vi "GeoData.vi"() -> ()   [LabVIEW 2017] (continued)
County\tH1\n43768\t39059\tOld washington\tOH\tGuernsey County\tH1\n43732\t39059\tCumberland\tOH\tGuernsey County\tH1\n43778\t39059\tSalesville\tOH\tGuernsey County\tH1\n43713\t39059\tBarnesville\tOH\tGuernsey County\tH1\n43722\t39059\tBuffalo\tOH\tGuernsey County\tH1\n43736\t39059\tFairview\tOH\tGuernsey County\tH1\n45013\t39061\tHamilton\tOH\tHamilton County\tH1\n45014\t39061\tFairfield\tOH\tHamilton County\tH1\n45002\t39061\tCleves\tOH\tHamilton County\tH1\n45236\t39061\tCincinnati\tOH\tHamilton County\tH1\n45248\t39061\tCincinnati\tOH\tHamilton County\tH1\n45255\t39061\tCincinnati\tOH\tHamilton County\tH1\n45249\t39061\tCincinnati\tOH\tHamilton County\tH1\n45253\t39061\tCincinnati\tOH\tHamilton County\tH1\n45262\t39061\tCincinnati\tOH\tHamilton County\tH1\n45258\t39061\tCincinnati\tOH\tHamilton County\tH1\n45041\t39061\tMiamitown\tOH\tHamilton County\tH1\n45150\t39061\tMilford\tOH\tHamilton County\tH1\n45069\t39061\tWest chester\tOH\tHamilton County\tH1\n45201\t39061\tCincinnati\tOH\tHamilton County\tH1\n45233\t39061\tCincinnati\tOH\tHamilton County\tH1\n45219\t39061\tCincinnati\tOH\tHamilton County\tH1\n45254\t39061\tCincinnati\tOH\tHamilton County\tH1\n45111\t39061\tCamp dennison\tOH\tHamilton County\tH1\n45263\t39061\tCincinnati\tOH\tHamilton County\tH1\n45208\t39061\tCincinnati\tOH\tHamilton County\tH1\n45211\t39061\tCincinnati\tOH\tHamilton County\tH1\n45204\t39061\tCincinnati\tOH\tHamilton County\tH1\n45226\t39061\tCincinnati\tOH\tHamilton County\tH1\n45227\t39061\tCincinnati\tOH\tHamilton County\tH1\n45229\t39061\tCincinnati\tOH\tHamilton County\tH1\n45220\t39061\tCincinnati\tOH\tHamilton County\tH1\n45235\t39061\tCincinnati\tOH\tHamilton County\tH1\n45030\t39061\tHarrison\tOH\tHamilton County\tH1\n45033\t39061\tHooven\tOH\tHamilton County\tH1\n45206\t39061\tCincinnati\tOH\tHamilton County\tH1\n45212\t39061\tCincinnati\tOH\tHamilton County\tH1\n45213\t39061\tCincinnati\tOH\tHamilton County\tH1\n45247\t39061\tCincinnati\tOH\tHamilton County\tH1\n45224\t39061\tCincinnati\tOH\tHamilton County\tH1\n45238\t39061\tCincinnati\tOH\tHamilton County\tH1\n45230\t39061\tCincinnati\tOH\tHamilton County\tH1\n45052\t39061\tNorth bend\tOH\tHamilton County\tH1\n45202\t39061\tCincinnati\tOH\tHamilton County\tH1\n45215\t39061\tCincinnati\tOH\tHamilton County\tH1\n45242\t39061\tCincinnati\tOH\tHamilton County\tH1\n45251\t39061\tCincinnati\tOH\tHamilton County\tH1\n45217\t39061\tCincinnati\tOH\tHamilton County\tH1\n45232\t39061\tCincinnati\tOH\tHamilton County\tH1\n45001\t39061\tAddyston\tOH\tHamilton County\tH1\n45222\t39061\tCincinnati\tOH\tHamilton County\tH1\n45209\t39061\tCincinnati\tOH\tHamilton County\tH1\n45216\t39061\tCincinnati\tOH\tHamilton County\tH1\n45239\t39061\tCincinnati\tOH\tHamilton County\tH1\n45244\t39061\tCincinnati\tOH\tHamilton County\tH1\n45231\t39061\tCincinnati\tOH\tHamilton County\tH1\n45252\t39061\tCincinnati\tOH\tHamilton County\tH1\n45223\t39061\tCincinnati\tOH\tHamilton County\tH1\n45225\t39061\tCincinnati\tOH\tHamilton County\tH1\n45250\t39061\tCincinnati\tOH\tHamilton County\tH1\n45218\t39061\tCincinnati\tOH\tHamilton County\tH1\n45234\t39061\tCincinnati\tOH\tHamilton County\tH1\n45203\t39061\tCincinnati\tOH\tHamilton County\tH1\n45246\t39061\tCincinnati\tOH\tHamilton County\tH1\n45237\t39061\tCincinnati\tOH\tHamilton County\tH1\n45243\t39061\tCincinnati\tOH\tHamilton County\tH1\n45267\t39061\tCincinnati\tOH\tHamilton County\tH1\n45140\t39061\tLoveland\tOH\tHamilton County\tH1\n45214\t39061\tCincinnati\tOH\tHamilton County\tH1\n45207\t39061\tCincinnati\tOH\tHamilton County\tH1\n45205\t39061\tCincinnati\tOH\tHamilton County\tH1\n45240\t39061\tCincinnati\tOH\tHamilton County\tH1\n45241\t39061\tCincinnati\tOH\tHamilton County\tH1\n45174\t39061\tTerrace park\tOH\tHamilton County\tH1\n45051\t39061\tMount saint joseph\tOH\tHamilton County\tH1\n45810\t39063\tAda\tOH\tHancock County\tH1\n45843\t39063\tForest\tOH\tHancock County\tH1\n45858\t39063\tMc comb\tOH\tHancock County\tH1\n45840\t39063\tFindlay\tOH\tHancock County\tH1\n45867\t39063\tMount blanchard\tOH\tHancock County\tH1\n45877\t39063\tPandora\tOH\tHancock County\tH1\n44802\t39063\tAlvada\tOH\tHancock County\tH1\n43516\t39063\tDeshler\tOH\tHancock County\tH1\n45814\t39063\tArlington\tOH\tHancock County\tH1\n45856\t39063\tLeipsic\tOH\tHancock County\tH1\n45881\t39063\tRawson\tOH\tHancock County\tH1\n44830\t39063\tFostoria\tOH\tHancock County\tH1\n45890\t39063\tVanlue\tOH\tHancock County\tH1\n45817\t39063\tBluffton\tOH\tHancock County\tH1\n45872\t39063\tNorth baltimore\tOH\tHancock County\tH1\n45836\t39063\tDunkirk\tOH\tHancock County\tH1\n45889\t39063\tVan buren\tOH\tHancock County\tH1\n45868\t39063\tMount cory\tOH\tHancock County\tH1\n44817\t39063\tBloomdale\tOH\tHancock County\tH1\n45841\t39063\tJenera\tOH\tHancock County\tH1\n43316\t39063\tCarey\tOH\tHancock County\tH1\n44804\t39063\tArcadia\tOH\tHancock County\tH1\n45839\t39063\tFindlay\tOH\tHancock County\tH1\n45897\t39063\tWilliamstown\tOH\tHancock County\tH1\n45816\t39063\tBenton ridge\tOH\tHancock County\tH1\n45810\t39065\tAda\tOH\tHardin County\tH1\n45843\t39065\tForest\tOH\tHardin County\tH1\n43331\t39065\tLakeview\tOH\tHardin County\tH1\n45850\t39065\tHarrod\tOH\tHardin County\tH1\n43345\t39065\tRidgeway\tOH\tHardin County\tH1\n43310\t39065\tBelle center\tOH\tHardin County\tH1\n43326\t39065\tKenton\tOH\tHardin County\tH1\n43332\t39065\tLa rue\tOH\tHardin County\tH1\n45896\t39065\tWaynesfield\tOH\tHardin County\tH1\n43340\t39065\tMount victory\tOH\tHardin County\tH1\n43347\t39065\tRushsylvania\tOH\tHardin County\tH1\n45859\t39065\tMc guffey\tOH\tHardin County\tH1\n45836\t39065\tDunkirk\tOH\tHardin County\tH1\n45835\t39065\tDola\tOH\tHardin County\tH1\n45841\t39065\tJenera\tOH\tHardin County\tH1\n43346\t39065\tRoundhead\tOH\tHardin County\tH1\n45812\t39065\tAlger\tOH\tHardin County\tH1\n44695\t39067\tBowerston\tOH\tHarrison County\tH1\n43977\t39067\tFlushing\tOH\tHarrison County\tH1\n44699\t39067\tTippecanoe\tOH\tHarrison County\tH1\n43976\t39067\tHopedale\tOH\tHarrison County\tH1\n43988\t39067\tScio\tOH\tHarrison County\tH1\n43907\t39067\tCadiz\tOH\tHarrison County\tH1\n44621\t39067\tDennison\tOH\tHarrison County\tH1\n43983\t39067\tPiedmont\tOH\tHarrison County\tH1\n43974\t39067\tHarrisville\tOH\tHarrison County\tH1\n43981\t39067\tNew athens\tOH\tHarrison County\tH1\n43984\t39067\tNew rumley\tOH\tHarrison County\tH1\n43901\t39067\tAdena\tOH\tHarrison County\tH1\n43973\t39067\tFreeport\tOH\tHarrison County\tH1\n44683\t39067\tUhrichsville\tOH\tHarrison County\tH1\n43986\t39067\tJewett\tOH\tHarrison County\tH1\n44693\t39067\tDeersville\tOH\tHarrison County\tH1\n43950\t39067\tSaint clairsville\tOH\tHarrison County\tH1\n43910\t39067\tBloomingdale\tOH\tHarrison County\tH1\n43527\t39069\tHolgate\tOH\tHenry County\tH1\n43532\t39069\tLiberty center\tOH\tHenry County\tH1\n43548\t39069\tNew bavaria\tOH\tHenry County\tH1\n43510\t39069\tColton\tOH\tHenry County\tH1\n43529\t39069\tHoytville\tOH\tHenry County\tH1\n43515\t39069\tDelta\tOH\tHenry County\tH1\n43516\t39069\tDeshler\tOH\tHenry County\tH1\n43524\t39069\tHamler\tOH\tHenry County\tH1\n45856\t39069\tLeipsic\tOH\tHenry County\tH1\n43535\t39069\tMalinta\tOH\tHenry County\tH1\n43523\t39069\tGrelton\tOH\tHenry County\tH1\n43567\t39069\tWauseon\tOH\tHenry County\tH1\n43512\t39069\tDefiance\tOH\tHenry County\tH1\n43522\t39069\tGrand rapids\tOH\tHenry County\tH1\n43534\t39069\tMc clure\tOH\tHenry County\tH1\n43555\t39069\tRidgeville corners\tOH\tHenry County\tH1\n43502\t39069\tArchbold\tOH\tHenry County\tH1\n43557\t39069\tStryker\tOH\tHenry County\tH1\n43545\t39069\tNapoleon\tOH\tHenry County\tH1\n43511\t39069\tCustar\tOH\tHenry County\tH1\n45660\t39071\tPeebles\tOH\tHighland County\tH1\n45118\t39071\tFayetteville\tOH\tHighland County\tH1\n45172\t39071\tSinking spring\tOH\tHighland County\tH1\n45142\t39071\tLynchburg\tOH\tHighland County\tH1\n45159\t39071\tNew vienna\tOH\tHighland County\tH1\n45697\t39071\tWinchester\tOH\tHighland County\tH1\n45154\t39071\tMount orab\tOH\tHighland County\tH1\n45132\t39071\tHighland\tOH\tHighland County\tH1\n45155\t39071\tMowrystown\tOH\tHighland County\tH1\n45171\t39071\tSardinia\tOH\tHighland County\tH1\n45123\t39071\tGreenfield\tOH\tHighland County\tH1\n45135\t39071\tLeesburg\tOH\tHighland County\tH1\n45679\t39071\tSeaman\tOH\tHighland County\tH1\n45133\t39071\tHillsboro\tOH\tHighland County\tH1\n45612\t39071\tBainbridge\tOH\tHighland County\tH1\n45654\t39073\tNew plymouth\tOH\tHocking County\tH1\n43158\t39073\tUnion furnace\tOH\tHocking County\tH1\n43155\t39073\tSugar grove\tOH\tHocking County\tH1\n43766\t39073\tNew straitsville\tOH\tHocking County\tH1\n43107\t39073\tBremen\tOH\tHocking County\tH1\n45622\t39073\tCreola\tOH\tHocking County\tH1\n43149\t39073\tRockbridge\tOH\tHocking County\tH1\n43102\t39073\tAmanda\tOH\tHocking County\tH1\n45732\t39073\tGlouster\tOH\tHocking County\tH1\n43127\t39073\tHaydenville\tOH\tHocking County\tH1\n43144\t39073\tMurray city\tOH\tHocking County\tH1\n43130\t39073\tLancaster\tOH\tHocking County\tH1\n43138\t39073\tLogan\tOH\tHocking County\tH1\n45764\t39073\tNelsonville\tOH\tHocking County\tH1\n43111\t39073\tCarbon hill\tOH\tHocking County\tH1\n43152\t39073\tSouth bloomingville\tOH\tHocking County\tH1\n43135\t39073\tLaurelville\tOH\tHocking County\tH1\n44660\t39075\tMount hope\tOH\tHolmes County\tH1\n44661\t39075\tNashville\tOH\tHolmes County\tH1\n44617\t39075\tCharm\tOH\tHolmes County\tH1\n44627\t39075\tFredericksburg\tOH\tHolmes County\tH1\n44690\t39075\tWinesburg\tOH\tHolmes County\tH1\n44637\t39075\tKillbuck\tOH\tHolmes County\tH1\n44610\t39075\tBerlin\tOH\tHolmes County\tH1\n44681\t39075\tSugarcreek\tOH\tHolmes County\tH1\n44676\t39075\tShreve\tOH\tHolmes County\tH1\n44689\t39075\tWilmot\tOH\tHolmes County\tH1\n44654\t39075\tMillersburg\tOH\tHolmes County\tH1\n44624\t39075\tDundee\tOH\tHolmes County\tH1\n43804\t39075\tBaltic\tOH\tHolmes County\tH1\n44628\t39075\tGlenmont\tOH\tHolmes County\tH1\n44687\t39075\tWalnut creek\tOH\tHolmes County\tH1\n44611\t39075\tBig prairie\tOH\tHolmes County\tH1\n44842\t39075\tLoudonville\tOH\tHolmes County\tH1\n43006\t39075\tBrinkhaven\tOH\tHolmes County\tH1\n44633\t39075\tHolmesville\tOH\tHolmes County\tH1\n44638\t39075\tLakeville\tOH\tHolmes County\tH1\n44847\t39077\tMonroeville\tOH\tHuron County\tH1\n44889\t39077\tWakeman\tOH\tHuron County\tH1\n44837\t39077\tGreenwich\tOH\tHuron County\tH1\n44878\t39077\tShiloh\tOH\tHuron County\tH1\n44826\t39077\tCollins\tOH\tHuron County\tH1\n44890\t39077\tWillard\tOH\tHuron County\tH1\n44851\t39077\tNew london\tOH\tHuron County\tH1\n44807\t39077\tAttica\tOH\tHuron County\tH1\n44811\t39077\tBellevue\tOH\tHuron County\tH1\n44865\t39077\tPlymouth\tOH\tHuron County\tH1\n44850\t39077\tNew haven\tOH\tHuron County\tH1\n44888\t39077\tWillard\tOH\tHuron County\tH1\n44855\t39077\tNorth fairfield\tOH\tHuron County\tH1\n44854\t39077\tNew washington\tOH\tHuron County\tH1\n44846\t39077\tMilan\tOH\tHuron County\tH1\n44857\t39077\tNorwalk\tOH\tHuron County\tH1\n45601\t39079\tChillicothe\tOH\tJackson County\tH1\n45621\t39079\tCoalton\tOH\tJackson County\tH1\n45653\t39079\tMinford\tOH\tJackson County\tH1\n45686\t39079\tVinton\tOH\tJackson County\tH1\n45656\t39079\tOak hill\tOH\tJackson County\tH1\n45634\t39079\tHamden\tOH\tJackson County\tH1\n45640\t39079\tJackson\tOH\tJackson County\tH1\n45672\t39079\tRay\tOH\tJackson County\tH1\n45682\t39079\tSouth webster\tOH\tJackson County\tH1\n45692\t39079\tWellston\tOH\tJackson County\tH1\n45685\t39079\tThurman\tOH\tJackson County\tH1\n45613\t39079\tBeaver\tOH\tJackson County\tH1\n43917\t39081\tDillonvale\tOH\tJefferson County\tH1\n43964\t39081\tToronto\tOH\tJefferson County\tH1\n43939\t39081\tMount pleasant\tOH\tJefferson County\tH1\n43943\t39081\tRayland\tOH\tJefferson County\tH1\n43907\t39081\tCadiz\tOH\tJefferson County\tH1\n43908\t39081\tBergholz\tOH\tJefferson County\tH1\n43944\t39081\tRichmond\tOH\tJefferson County\tH1\n43930\t39081\tHammondsville\tOH\tJefferson County\tH1\n43926\t39081\tEmpire\tOH\tJefferson County\tH1\n43945\t39081\tSalineville\tOH\tJefferson County\tH1\n43952\t39081\tSteubenville\tOH\tJefferson County\tH1\n43932\t39081\tIrondale\tOH\tJefferson County\tH1\n43963\t39081\tTiltonsville\tOH\tJefferson County\tH1\n43948\t39081\tSmithfield\tOH\tJefferson County\tH1\n43901\t39081\tAdena\tOH\tJefferson County\tH1\n43953\t39081\tSteubenville\tOH\tJefferson County\tH1\n43903\t39081\tAmsterdam\tOH\tJefferson County\tH1\n43941\t39081\tPiney fork\tOH\tJefferson County\tH1\n43925\t39081\tEast springfield\tOH\tJefferson County\tH1\n43938\t39081\tMingo junction\tOH\tJefferson County\tH1\n43971\t39081\tYorkville\tOH\tJefferson County\tH1\n43913\t39081\tBrilliant\tOH\tJefferson County\tH1\n43961\t39081\tStratton\tOH\tJefferson County\tH1\n43970\t39081\tWolf run\tOH\tJefferson County\tH1\n43910\t39081\tBloomingdale\tOH\tJefferson County\tH1\n43080\t39083\tUtica\tOH\tKnox County\tH1\n43050\t39083\tMount vernon\tOH\tKnox County\tH1\n44822\t39083\tButler\tOH\tKnox County\tH1\n43028\t39083\tHoward\tOH\tKnox County\tH1\n43022\t39083\tGambier\tOH\tKnox County\tH1\n44628\t39083\tGlenmont\tOH\tKnox County\tH1\n43005\t39083\tBladensburg\tOH\tKnox County\tH1\n44842\t39083\tLoudonville\tOH\tKnox County\tH1\n43844\t39083\tWarsaw\tOH\tKnox County\tH1\n43822\t39083\tFrazeysburg\tOH\tKnox County\tH1\n43006\t39083\tBrinkhaven\tOH\tKnox County\tH1\n43048\t39083\tMount liberty\tOH\tKnox County\tH1\n43014\t39083\tDanville\tOH\tKnox County\tH1\n43037\t39083\tMartinsburg\tOH\tKnox County\tH1\n44813\t39083\tBellville\tOH\tKnox County\tH1\n43019\t39083\tFredericktown\tOH\tKnox County\tH1\n43011\t39083\tCenterburg\tOH\tKnox County\tH1\n43843\t39083\tWalhonding\tOH\tKnox County\tH1\n44041\t39085\tGeneva\tOH\tLake County\tH1\n44086\t39085\tThompson\tOH\tLake County\tH1\n44024\t39085\tChardon\tOH\tLake County\tH1\n44060\t39085\tMentor\tOH\tLake County\tH1\n44094\t39085\tWilloughby\tOH\tLake County\tH1\n44092\t39085\tWickliffe\tOH\tLake County\tH1\n44095\t39085\tEastlake\tOH\tLake County\tH1\n44061\t39085\tMentor\tOH\tLake County\tH1\n44096\t39085\tWilloughby\tOH\tLake County\tH1\n44132\t39085\tEuclid\tOH\tLake County\tH1\n44057\t39085\tMadison\tOH\tLake County\tH1\n44081\t39085\tPerry\tOH\tLake County\tH1\n44077\t39085\tPainesville\tOH\tLake County\tH1\n44045\t39085\tGrand river\tOH\tLake County\tH1\n45623\t39087\tCrown city\tOH\tLawrence County\tH1\n45658\t39087\tPatriot\tOH\tLawrence County\tH1\n45638\t39087\tIronton\tOH\tLawrence County\tH1\n45669\t39087\tProctorville\tOH\tLawrence County\tH1\n45688\t39087\tWaterloo\tOH\tLawrence County\tH1\n45629\t39087\tFranklin furnace\tOH\tLawrence County\tH1\n45696\t39087\tWillow wood\tOH\tLawrence County\tH1\n45659\t39087\tPedro\tOH\tLawrence County\tH1\n45656\t39087\tOak hill\tOH\tLawrence County\tH1\n45645\t39087\tKitts hill\tOH\tLawrence County\tH1\n45619\t39087\tChesapeake\tOH\tLawrence County\tH1\n45682\t39087\tSouth webster\tOH\tLawrence County\tH1\n45675\t39087\tRock camp\tOH\tLawrence County\tH1\n45680\t39087\tSouth point\tOH\tLawrence County\tH1\n45678\t39087\tScottown\tOH\tLawrence County\tH1\n43076\t39089\tThornville\tOH\tLicking County\tH1\n43080\t39089\tUtica\tOH\tLicking County\tH1\n43050\t39089\tMount vernon\tOH\tLicking County\tH1\n43023\t39089\tGranville\tOH\tLicking County\tH1\n43746\t39089\tHopewell\tOH\tLicking County\tH1\n43031\t39089\tJohnstown\tOH\tLicking County\tH1\n43739\t39089\tGlenford\tOH\tLicking County\tH1\n43004\t39089\tBlacklick\tOH\tLicking County\tH1\n43018\t39089\tEtna\tOH\tLicking County\tH1\n43760\t39089\tMount perry\tOH\tLicking County\tH1\n43030\t39089\tJacksontown\tOH\tLicking County\tH1\n43105\t39089\tBaltimore\tOH\tLicking County\tH1\n43147\t39089\tPickerington\tOH\tLicking County\tH1\n43740\t39089\tGratiot\tOH\tLicking County\tH1\n43054\t39089\tNew albany\tOH\tLicking County\tH1\n43046\t39089\tMillersport\tOH\tLicking County\tH1\n43830\t39089\tNashport\tOH\tLicking County\tH1\n43025\t39089\tHebron\tOH\tLicking County\tH1\n43033\t39089\tKirkersville\tOH\tLicking County\tH1\n43068\t39089\tReynoldsburg\tOH\tLicking County\tH1\n43055\t39089\tNewark\tOH\tLicking County\tH1\n43056\t39089\tHeath\tOH\tLicking County\tH1\n43013\t39089\tCroton\tOH\tLicking County\tH1\n43822\t39089\tFrazeysburg\tOH\tLicking County\tH1\n43027\t39089\tHomer\tOH\tLicking County\tH1\n43071\t39089\tSaint louisville\tOH\tLicking County\tH1\n43074\t39089\tSunbury\tOH\tLicking County\tH1\n43062\t39089\tPataskala\tOH\tLicking County\tH1\n43008\t39089\tBuckeye lake\tOH\tLicking County\tH1\n43058\t39089\tNewark\tOH\tLicking County\tH1\n43011\t39089\tCenterburg\tOH\tLicking County\tH1\n43001\t39089\tAlexandria\tOH\tLicking County\tH1\n43721\t39089\tBrownsville\tOH\tLicking County\tH1\n43073\t39089\tSummit station\tOH\tLicking County\tH1\n43331\t39091\tLakeview\tOH\tLogan County\tH1\n43311\t39091\tBellefontaine\tOH\tLogan County\tH1\n43319\t39091\tEast liberty\tOH\tLogan County\tH1\n43348\t39091\tRussells point\tOH\tLogan County\tH1\n43345\t39091\tRidgeway\tOH\tLogan County\tH1\n43310\t39091\tBelle center\tOH\tLogan County\tH1\n43357\t39091\tWest liberty\tOH\tLogan County\tH1\n43067\t39091\tRaymond\tOH\tLogan County\tH1\n45895\t39091\tWapakoneta\tOH\tLogan County\tH1\n43060\t39091\tNorth lewisburg\tOH\tLogan County\tH1\n43347\t39091\tRushsylvania\tOH\tLogan County\tH1\n43336\t39091\tMiddleburg\tOH\tLogan County\tH1\n43358\t39091\tWest mansfield\tOH\tLogan County\tH1\n43333\t39091\tLewistown\tOH\tLogan County\tH1\n43343\t39091\tQuincy\tOH\tLogan County\tH1\n43318\t39091\tDe graff\tOH\tLogan County\tH1\n43360\t39091\tZanesfield\tOH\tLogan County\tH1\n45334\t39091\tJackson center\tOH\tLogan County\tH1\n43324\t39091\tHuntsville\tOH\tLogan County\tH1\n44275\t39093\tSpencer\tOH\tLorain County\tH1\n44074\t39093\tOberlin\tOH\tLorain County\tH1\n44859\t39093\tNova\tOH\tLorain County\tH1\n44012\t39093\tAvon lake\tOH\tLorain County\tH1\n44256\t39093\tMedina\tOH\tLorain County\tH1\n44889\t39093\tWakeman\tOH\tLorain County\tH1\n44044\t39093\tGrafton\tOH\tLorain County\tH1\n44039\t39093\tNorth ridgeville\tOH\tLorain County\tH1\n44001\t39093\tAmherst\tOH\tLorain County\tH1\n44052\t39093\tLorain\tOH\tLorain County\tH1\n44851\t39093\tNew london\tOH\tLorain County\tH1\n44049\t39093\tKipton\tOH\tLorain County\tH1\n44011\t39093\tAvon\tOH\tLorain County\tH1\n44280\t39093\tValley city\tOH\tLorain County\tH1\n44090\t39093\tWellington\tOH\tLorain County\tH1\n44880\t39093\tSullivan\tOH\tLorain County\tH1\n44036\t39093\tElyria\tOH\tLorain County\tH1\n44035\t39093\tElyria\tOH\tLorain County\tH1\n44053\t39093\tLorain\tOH\tLorain County\tH1\n44028\t39093\tColumbia station\tOH\tLorain County\tH1\n44253\t39093\tLitchfield\tOH\tLorain County\tH1\n44089\t39093\tVermilion\tOH\tLorain County\tH1\n44054\t39093\tSheffield lake\tOH\tLorain County\tH1\n44050\t39093\tLagrange\tOH\tLorain County\tH1\n44055\t39093\tLorain\tOH\tLorain County\tH1\n43612\t39095\tToledo\tOH\tLucas County\tH1\n43606\t39095\tToledo\tOH\tLucas County\tH1\n43571\t39095\tWhitehouse\tOH\tLucas County\tH1\n43609\t39095\tToledo\tOH\tLucas County\tH1\n43532\t39095\tLiberty center\tOH\tLucas County\tH1\n43504\t39095\tBerkey\tOH\tLucas County\tH1\n43547\t39095\tNeapolis\tOH\tLucas County\tH1\n43434\t39095\tHarbor view\tOH\tLucas County\tH1\n43615\t39095\tToledo\tOH\tLucas County\tH1\n43623\t39095\tToledo\tOH\tLucas County\tH1\n43560\t39095\tSylvania\tOH\tLucas County\tH1\n43619\t39095\tNorthwood\tOH\tLucas County\tH1\n43537\t39095\tMaumee\tOH\tLucas County\tH1\n43445\t39095\tMartin\tOH\tLucas County\tH1\n43601\t39095\tToledo\tOH\tLucas County\tH1\n43656\t39095\tToledo\tOH\tLucas County\tH1\n43558\t39095\tSwanton\tOH\tLucas County\tH1\n43528\t39095\tHolland\tOH\tLucas County\tH1\n43635\t39095\tToledo\tOH\tLucas County\tH1\n43659\t39095\tToledo\tOH\tLucas County\tH1\n43657\t39095\tToledo\tOH\tLucas County\tH1\n43611\t39095\tToledo\tOH\tLucas County\tH1\n43614\t39095\tToledo\tOH\tLucas County\tH1\n43604\t39095\tToledo\tOH\tLucas County\tH1\n43666\t39095\tToledo\tOH\tLucas County\tH1\n43667\t39095\tToledo\tOH\tLucas County\tH1\n43613\t39095\tToledo\tOH\tLucas County\tH1\n43620\t39095\tToledo\tOH\tLucas County\tH1\n43617\t39095\tToledo\tOH\tLucas County\tH1\n43412\t39095\tCurtice\tOH\tLucas County\tH1\n43522\t39095\tGrand rapids\tOH\tLucas County\tH1\n43661\t39095\tToledo\tOH\tLucas County\tH1\n43605\t39095\tToledo\tOH\tLucas County\tH1\n43607\t39095\tToledo\tOH\tLucas County\tH1\n43616\t39095\tOregon\tOH\tLucas County\tH1\n43566\t39095\tWaterville\tOH\tLucas County\tH1\n43608\t39095\tToledo\tOH\tLucas County\tH1\n45348\t39095\tNew weston\tOH\tLucas County\tH1\n43660\t39095\tToledo\tOH\tLucas County\tH1\n43652\t39095\tToledo\tOH\tLucas County\tH1\n43542\t39095\tMonclova\tOH\tLucas County\tH1\n43610\t39095\tToledo\tOH\tLucas County\tH1\n43064\t39097\tPlain city\tOH\tMadison County\tH1\n43026\t39097\tHilliard\tOH\tMadison County\tH1\n43029\t39097\tIrwin\tOH\tMadison County\tH1\n45369\t39097\tSouth vienna\tOH\tMadison County\tH1\n43151\t39097\tSedalia\tOH\tMadison County\tH1\n43123\t39097\tGrove city\tOH\tMadison County\tH1\n43162\t39097\tWest jefferson\tOH\tMadison County\tH1\n43140\t39097\tLondon\tOH\tMadison County\tH1\n43143\t39097\tMount sterling\tOH\tMadison County\tH1\n43153\t39097\tSouth solon\tOH\tMadison County\tH1\n43119\t39097\tGalloway\tOH\tMadison County\tH1\n43044\t39097\tMechanicsburg\tOH\tMadison County\tH1\n43146\t39097\tOrient\tOH\tMadison County\tH1\n44512\t39099\tYoungstown\tOH\tMahoning County\tH1\n44451\t39099\tNorth jackson\tOH\tMahoning County\tH1\n44501\t39099\tYoungstown\tOH\tMahoning County\tH1\n44449\t39099\tNorth benton\tOH\tMahoning County\tH1\n44454\t39099\tPetersburg\tOH\tMahoning County\tH1\n44416\t39099\tEllsworth\tOH\tMahoning County\tH1\n44437\t39099\tMc donald\tOH\tMahoning County\tH1\n44460\t39099\tSalem\tOH\tMahoning County\tH1\n44408\t39099\tColumbiana\tOH\tMahoning County\tH1\n44511\t39099\tYoungstown\tOH\tMahoning County\tH1\n44514\t39099\tYoungstown\tOH\tMahoning County\tH1\n44452\t39099\tNorth lima\tOH\tMahoning County\tH1\n44405\t39099\tCampbell\tOH\tMahoning County\tH1\n44504\t39099\tYoungstown\tOH\tMahoning County\tH1\n44436\t39099\tLowellville\tOH\tMahoning County\tH1\n44506\t39099\tYoungstown\tOH\tMahoning County\tH1\n44422\t39099\tGreenford\tOH\tMahoning County\tH1\n44471\t39099\tStruthers\tOH\tMahoning County\tH1\n44507\t39099\tYoungstown\tOH\tMahoning County\tH1\n44503\t39099\tYoungstown\tOH\tMahoning County\tH1\n44481\t39099\tWarren\tOH\tMahoning County\tH1\n44406\t39099\tCanfield\tOH\tMahoning County\tH1\n44515\t39099\tYoungstown\tOH\tMahoning County\tH1\n44509\t39099\tYoungstown\tOH\tMahoning County\tH1\n44490\t39099\tWashingtonville\tOH\tMahoning County\tH1\n44443\t39099\tNew springfield\tOH\tMahoning County\tH1\n44442\t39099\tNew middletown\tOH\tMahoning County\tH1\n44601\t39099\tAlliance\tOH\tMahoning County\tH1\n44672\t39099\tSebring\tOH\tMahoning County\tH1\n44510\t39099\tYoungstown\tOH\tMahoning County\tH1\n44513\t39099\tYoungstown\tOH\tMahoning County\tH1\n44412\t39099\tDiamond\tOH\tMahoning County\tH1\n44555\t39099\tYoungstown\tOH\tMahoning County\tH1\n44425\t39099\tHubbard\tOH\tMahoning County\tH1\n44440\t39099\tMineral ridge\tOH\tMahoning County\tH1\n44401\t39099\tBerlin center\tOH\tMahoning County\tH1\n44429\t39099\tLake milton\tOH\tMahoning County\tH1\n44502\t39099\tYoungstown\tOH\tMahoning County\tH1\n44505\t39099\tYoungstown\tOH\tMahoning County\tH1\n44619\t39099\tDamascus\tOH\tMahoning County\tH1\n44444\t39099\tNewton falls\tOH\tMahoning County\tH1\n44609\t39099\tBeloit\tOH\tMahoning County\tH1\n45843\t39101\tForest\tOH\tMarion County\tH1\n44849\t39101\tNevada\tOH\tMarion County\tH1\n43344\t39101\tRichwood\tOH\tMarion County\tH1\n43326\t39101\tKenton\tOH\tMarion County\tH1\n43332\t39101\tLa rue\tOH\tMarion County\tH1\n43314\t39101\tCaledonia\tOH\tMarion County\tH1\n43337\t39101\tMorral\tOH\tMarion County\tH1\n43302\t39101\tMarion\tOH\tMarion County\tH1\n43315\t39101\tCardington\tOH\tMarion County\tH1\n43341\t39101\tNew bloomington\tOH\tMarion County\tH1\n43322\t39101\tGreen camp\tOH\tMarion County\tH1\n43342\t39101\tProspect\tOH\tMarion County\tH1\n44833\t39101\tGalion\tOH\tMarion County\tH1\n43323\t39101\tHarpster\tOH\tMarion County\tH1\n43356\t39101\tWaldo\tOH\tMarion County\tH1\n44275\t39103\tSpencer\tOH\tMedina County\tH1\n44258\t39103\tMedina\tOH\tMedina County\tH1\n44256\t39103\tMedina\tOH\tMedina County\tH1\n44287\t39103\tWest salem\tOH\tMedina County\tH1\n44251\t39103\tWestfield center\tOH\tMedina County\tH1\n44235\t39103\tHomerville\tOH\tMedina County\tH1\n44215\t39103\tChippewa lake\tOH\tMedina County\tH1\n44274\t39103\tSharon center\tOH\tMedina County\tH1\n44233\t39103\tHinckley\tOH\tMedina County\tH1\n44217\t39103\tCreston\tOH\tMedina County\tH1\n44044\t39103\tGrafton\tOH\tMedina County\tH1\n44230\t39103\tDoylestown\tOH\tMedina County\tH1\n44212\t39103\tBrunswick\tOH\tMedina County\tH1\n44254\t39103\tLodi\tOH\tMedina County\tH1\n44273\t39103\tSeville\tOH\tMedina County\tH1\n44280\t39103\tValley city\tOH\tMedina County\tH1\n44090\t39103\tWellington\tOH\tMedina County\tH1\n44880\t39103\tSullivan\tOH\tMedina County\tH1\n44149\t39103\tStrongsville\tOH\tMedina County\tH1\n44214\t39103\tBurbank\tOH\tMedina County\tH1\n44281\t39103\tWadsworth\tOH\tMedina County\tH1\n44333\t39103\tAkron\tOH\tMedina County\tH1\n44321\t39103\tAkron\tOH\tMedina County\tH1\n44028\t39103\tColumbia station\tOH\tMedina County\tH1\n44203\t39103\tBarberton\tOH\tMedina County\tH1\n44270\t39103\tRittman\tOH\tMedina County\tH1\n44253\t39103\tLitchfield\tOH\tMedina County\tH1\n45723\t39105\tCoolville\tOH\tMeigs County\tH1\n45770\t39105\tPortland\tOH\tMeigs County\tH1\n45720\t39105\tChester\tOH\tMeigs County\tH1\n45776\t39105\tShade\tOH\tMeigs County\tH1\n45769\t39105\tPomeroy\tOH\tMeigs County\tH1\n45771\t39105\tRacine\tOH\tMeigs County\tH1\n45741\t39105\tLangsville\tOH\tMeigs County\tH1\n45760\t39105\tMiddleport\tOH\tMeigs County\tH1\n45614\t39105\tBidwell\tOH\tMeigs County\tH1\n45775\t39105\tRutland\tOH\tMeigs County\tH1\n45686\t39105\tVinton\tOH\tMeigs County\tH1\n45735\t39105\tGuysville\tOH\tMeigs County\tH1\n45783\t39105\tTuppers plains\tOH\tMeigs County\tH1\n45710\t39105\tAlbany\tOH\tMeigs County\tH1\n45743\t39105\tLong bottom\tOH\tMeigs County\tH1\n45772\t39105\tReedsville\tOH\tMeigs County\tH1\n45779\t39105\tSyracuse\tOH\tMeigs County\tH1\n45620\t39105\tCheshire\tOH\tMeigs County\tH1\n45865\t39107\tMinster\tOH\tMercer County\tH1\n45862\t39107\tMendon\tOH\tMercer County\tH1\n45860\t39107\tMaria stein\tOH\tMercer County\tH1\n45883\t39107\tSaint henry\tOH\tMercer County\tH1\n45882\t39107\tRockford\tOH\tMercer County\tH1\n45826\t39107\tChickasaw\tOH\tMercer County\tH1\n45822\t39107\tCelina\tOH\tMercer County\tH1\n45898\t39107\tWillshire\tOH\tMercer County\tH1\n45869\t39107\tNew bremen\tOH\tMercer County\tH1\n45388\t39107\tYorkshire\tOH\tMercer County\tH1\n45894\t39107\tVenedocia\tOH\tMercer County\tH1\n45885\t39107\tSaint marys\tOH\tMercer County\tH1\n45887\t39107\tSpencerville\tOH\tMercer County\tH1\n45846\t39107\tFort recovery\tOH\tMercer County\tH1\n45348\t39107\tNew weston\tOH\tMercer County\tH1\n45828\t39107\tColdwater\tOH\tMercer County\tH1\n45845\t39107\tFort loramie\tOH\tMercer County\tH1\n45310\t39107\tBurkettsville\tOH\tMercer County\tH1\n45866\t39107\tMontezuma\tOH\tMercer County\tH1\n45371\t39109\tTipp city\tOH\tMiami County\tH1\n45383\t39109\tWest milton\tOH\tMiami County\tH1\n45361\t39109\tPotsdam\tOH\tMiami County\tH1\n45374\t39109\tTroy\tOH\tMiami County\tH1\n45304\t39109\tArcanum\tOH\tMiami County\tH1\n45337\t39109\tLaura\tOH\tMiami County\tH1\n45326\t39109\tFletcher\tOH\tMiami County\tH1\n45317\t39109\tConover\tOH\tMiami County\tH1\n45318\t39109\tCovington\tOH\tMiami County\tH1\n45424\t39109\tDayton\tOH\tMiami County\tH1\n45308\t39109\tBradford\tOH\tMiami County\tH1\n45322\t39109\tEnglewood\tOH\tMiami County\tH1\n45344\t39109\tNew carlisle\tOH\tMiami County\tH1\n45339\t39109\tLudlow falls\tOH\tMiami County\tH1\n45373\t39109\tTroy\tOH\tMiami County\tH1\n45365\t39109\tSidney\tOH\tMiami County\tH1\n45312\t39109\tCasstown\tOH\tMiami County\tH1\n45356\t39109\tPiqua\tOH\tMiami County\tH1\n45359\t39109\tPleasant hill\tOH\tMiami County\tH1\n43793\t39111\tWoodsfield\tOH\tMonroe County\tH1\n43942\t39111\tPowhatan point\tOH\tMonroe County\tH1\n43946\t39111\tSardis\tOH\tMonroe County\tH1\n43754\t39111\tLewisville\tOH\tMonroe County\tH1\n43915\t39111\tClarington\tOH\tMonroe County\tH1\n43716\t39111\tBeallsville\tOH\tMonroe County\tH1\n45767\t39111\tNew matamoras\tOH\tMonroe County\tH1\n45734\t39111\tGraysville\tOH\tMonroe County\tH1\n43914\t39111\tCameron\tOH\tMonroe County\tH1\n43773\t39111\tQuaker city\tOH\tMonroe County\tH1\n43747\t39111\tJerusalem\tOH\tMonroe County\tH1\n43788\t39111\tSummerfield\tOH\tMonroe County\tH1\n45745\t39111\tLower salem\tOH\tMonroe County\tH1\n43786\t39111\tStafford\tOH\tMonroe County\tH1\n43752\t39111\tLaings\tOH\tMonroe County\tH1\n43931\t39111\tHannibal\tOH\tMonroe County\tH1\n43757\t39111\tMalaga\tOH\tMonroe County\tH1\n45789\t39111\tWingett run\tOH\tMonroe County\tH1\n45005\t39113\tFranklin\tOH\tMontgomery County\tH1\n45342\t39113\tMiamisburg\tOH\tMontgomery County\tH1\n45315\t39113\tClayton\tOH\tMontgomery County\tH1\n45371\t39113\tTipp city\tOH\tMontgomery County\tH1\n45440\t39113\tDayton\tOH\tMontgomery County\tH1\n45430\t39113\tDayton\tOH\tMontgomery County\tH1\n45345\t39113\tNew lebanon\tOH\tMontgomery County\tH1\n45343\t39113\tMiamisburg\tOH\tMontgomery County\tH1\n45490\t39113\tDayton\tOH\tMontgomery County\tH1\n45354\t39113\tPhillipsburg\tOH\tMontgomery County\tH1\n45377\t39113\tVandalia\tOH\tMontgomery County\tH1\n45415\t39113\tDayton\tOH\tMontgomery County\tH1\n45401\t39113\tDayton\tOH\tMontgomery County\tH1\n45439\t39113\tDayton\tOH\tMontgomery County\tH1\n45416\t39113\tDayton\tOH\tMontgomery County\tH1\n45428\t39113\tDayton\tOH\tMontgomery County\tH1\n45066\t39113\tSpringboro\tOH\tMontgomery County\tH1\n45338\t39113\tLewisburg\tOH\tMontgomery County\tH1\n45409\t39113\tDayton\tOH\tMontgomery County\tH1\n45433\t39113\tDayton\tOH\tMontgomery County\tH1\n45309\t39113\tBrookville\tOH\tMontgomery County\tH1\n45327\t39113\tGermantown\tOH\tMontgomery County\tH1\n45403\t39113\tDayton\tOH\tMontgomery County\tH1\n45406\t39113\tDayton\tOH\tMontgomery County\tH1\n45429\t39113\tDayton\tOH\tMontgomery County\tH1\n45381\t39113\tWest alexandria\tOH\tMontgomery County\tH1\n45423\t39113\tDayton\tOH\tMontgomery County\tH1\n45422\t39113\tDayton\tOH\tMontgomery County\tH1\n45417\t39113\tDayton\tOH\tMontgomery County\tH1\n45419\t39113\tDayton\tOH\tMontgomery County\tH1\n45424\t39113\tDayton\tOH\tMontgomery County\tH1\n45431\t39113\tDayton\tOH\tMontgomery County\tH1\n45449\t39113\tDayton\tOH\tMontgomery County\tH1\n45322\t39113\tEnglewood\tOH\tMontgomery County\tH1\n45405\t39113\tDayton\tOH\tMontgomery County\tH1\n45414\t39113\tDayton\tOH\tMontgomery County\tH1\n45344\t39113\tNew carlisle\tOH\tMontgomery County\tH1\n45420\t39113\tDayton\tOH\tMontgomery County\tH1\n45378\t39113\tVerona\tOH\tMontgomery County\tH1\n45042\t39113\tMiddletown\tOH\tMontgomery County\tH1\n45402\t39113\tDayton\tOH\tMontgomery County\tH1\n45404\t39113\tDayton\tOH\tMontgomery County\tH1\n45410\t39113\tDayton\tOH\tMontgomery County\tH1\n45426\t39113\tDayton\tOH\tMontgomery County\tH1\n45413\t39113\tDayton\tOH\tMontgomery County\tH1\n45458\t39113\tDayton\tOH\tMontgomery County\tH1\n45475\t39113\tDayton\tOH\tMontgomery County\tH1\n45437\t39113\tDayton\tOH\tMontgomery County\tH1\n45469\t39113\tDayton\tOH\tMontgomery County\tH1\n45470\t39113\tDayton\tOH\tMontgomery County\tH1\n45448\t39113\tDayton\tOH\tMontgomery County\tH1\n45325\t39113\tFarmersville\tOH\tMontgomery County\tH1\n45432\t39113\tDayton\tOH\tMontgomery County\tH1\n45441\t39113\tDayton\tOH\tMontgomery County\tH1\n45459\t39113\tDayton\tOH\tMontgomery County\tH1\n43787\t39115\tStockport\tOH\tMorgan County\tH1\n45715\t39115\tBeverly\tOH\tMorgan County\tH1\n43777\t39115\tRoseville\tOH\tMorgan County\tH1\n45744\t39115\tLowell\tOH\tMorgan County\tH1\n43724\t39115\tCaldwell\tOH\tMorgan County\tH1\n45711\t39115\tAmesville\tOH\tMorgan County\tH1\n43756\t39115\tMcconnelsville\tOH\tMorgan County\tH1\n45732\t39115\tGlouster\tOH\tMorgan County\tH1\n45786\t39115\tWaterford\tOH\tMorgan County\tH1\n43758\t39115\tMalta\tOH\tMorgan County\tH1\n43720\t39115\tBlue rock\tOH\tMorgan County\tH1\n43728\t39115\tChesterhill\tOH\tMorgan County\tH1\n43731\t39115\tCrooksville\tOH\tMorgan County\tH1\n43050\t39117\tMount vernon\tOH\tMorrow County\tH1\n43334\t39117\tMarengo\tOH\tMorrow County\tH1\n43350\t39117\tSparta\tOH\tMorrow County\tH1\n44903\t39117\tMansfield\tOH\tMorrow County\tH1\n43314\t39117\tCaledonia\tOH\tMorrow County\tH1\n43317\t39117\tChesterville\tOH\tMorrow County\tH1\n44904\t39117\tMansfield\tOH\tMorrow County\tH1\n43315\t39117\tCardington\tOH\tMorrow County\tH1\n43320\t39117\tEdison\tOH\tMorrow County\tH1\n43321\t39117\tFulton\tOH\tMorrow County\tH1\n43349\t39117\tShauck\tOH\tMorrow County\tH1\n43338\t39117\tMount gilead\tOH\tMorrow County\tH1\n44833\t39117\tGalion\tOH\tMorrow County\tH1\n43003\t39117\tAshley\tOH\tMorrow County\tH1\n43325\t39117\tIberia\tOH\tMorrow County\tH1\n44813\t39117\tBellville\tOH\tMorrow County\tH1\n43019\t39117\tFredericktown\tOH\tMorrow County\tH1\n43011\t39117\tCenterburg\tOH\tMorrow County\tH1\n43356\t39117\tWaldo\tOH\tMorrow County\tH1\n43746\t39119\tHopewell\tOH\tMuskingum County\tH1\n43777\t39119\tRoseville\tOH\tMuskingum County\tH1\n43791\t39119\tWhite cottage\tOH\tMuskingum County\tH1\n43821\t39119\tDresden\tOH\tMuskingum County\tH1\n43760\t39119\tMount perry\tOH\tMuskingum County\tH1\n43762\t39119\tNew concord\tOH\tMuskingum County\tH1\n43811\t39119\tConesville\tOH\tMuskingum County\tH1\n43842\t39119\tTrinway\tOH\tMuskingum County\tH1\n43771\t39119\tPhilo\tOH\tMuskingum County\tH1\n43756\t39119\tMcconnelsville\tOH\tMuskingum County\tH1\n43830\t39119\tNashport\tOH\tMuskingum County\tH1\n43056\t39119\tHeath\tOH\tMuskingum County\tH1\n43734\t39119\tDuncan falls\tOH\tMuskingum County\tH1\n43767\t39119\tNorwich\tOH\tMuskingum County\tH1\n43727\t39119\tChandlersville\tOH\tMuskingum County\tH1\n43720\t39119\tBlue rock\tOH\tMuskingum County\tH1\n43822\t39119\tFrazeysburg\tOH\tMuskingum County\tH1\n43701\t39119\tZanesville\tOH\tMuskingum County\tH1\n43732\t39119\tCumberland\tOH\tMuskingum County\tH1\n43702\t39119\tZanesville\tOH\tMuskingum County\tH1\n43735\t39119\tEast fultonham\tOH\tMuskingum County\tH1\n43738\t39119\tFultonham\tOH\tMuskingum County\tH1\n43802\t39119\tAdamsville\tOH\tMuskingum County\tH1\n43772\t39121\tPleasant city\tOH\tNoble County\tH1\n45715\t39121\tBeverly\tOH\tNoble County\tH1\n45727\t39121\tDexter city\tOH\tNoble County\tH1\n45746\t39121\tMacksburg\tOH\tNoble County\tH1\n45744\t39121\tLowell\tOH\tNoble County\tH1\n43724\t39121\tCaldwell\tOH\tNoble County\tH1\n43779\t39121\tSarahsville\tOH\tNoble County\tH1\n43717\t39121\tBelle valley\tOH\tNoble County\tH1\n43773\t39121\tQuaker city\tOH\tNoble County\tH1\n43788\t39121\tSummerfield\tOH\tNoble County\tH1\n45745\t39121\tLower salem\tOH\tNoble County\tH1\n43780\t39121\tSenecaville\tOH\tNoble County\tH1\n43711\t39121\tAva\tOH\tNoble County\tH1\n43732\t39121\tCumberland\tOH\tNoble County\tH1\n43778\t39121\tSalesville\tOH\tNoble County\tH1\n43713\t39121\tBarnesville\tOH\tNoble County\tH1\n43416\t39123\tElmore\tOH\tOttawa County\tH1\n43408\t39123\tClay center\tOH\tOttawa County\tH1\n43452\t39123\tPort clinton\tOH\tOttawa County\tH1\n43432\t39123\tGraytown\tOH\tOttawa County\tH1\n43440\t39123\tLakeside marblehead\tOH\tOttawa County\tH1\n43449\t39123\tOak harbor\tOH\tOttawa County\tH1\n43445\t39123\tMartin\tOH\tOttawa County\tH1\n43456\t39123\tPut in bay\tOH\tOttawa County\tH1\n43446\t39123\tMiddle bass\tOH\tOttawa County\tH1\n43447\t39123\tMillbury\tOH\tOttawa County\tH1\n43469\t39123\tWoodville\tOH\tOttawa County\tH1\n43412\t39123\tCurtice\tOH\tOttawa County\tH1\n43433\t39123\tGypsum\tOH\tOttawa County\tH1\n43458\t39123\tRocky ridge\tOH\tOttawa County\tH1\n43430\t39123\tGenoa\tOH\tOttawa County\tH1\n43468\t39123\tWilliston\tOH\tOttawa County\tH1\n43439\t39123\tLacarne\tOH\tOttawa County\tH1\n43420\t39123\tFremont\tOH\tOttawa County\tH1\n43442\t39123\tLindsey\tOH\tOttawa County\tH1\n43436\t39123\tIsle saint george\tOH\tOttawa County\tH1\n45832\t39125\tConvoy\tOH\tPaulding County\tH1\n45861\t39125\tMelrose\tOH\tPaulding County\tH1\n45873\t39125\tOakwood\tOH\tPaulding County\tH1\n45813\t39125\tAntwerp\tOH\tPaulding County\tH1\n45831\t39125\tContinental\tOH\tPaulding County\tH1\n45849\t39125\tGrover hill\tOH\tPaulding County\tH1\n45821\t39125\tCecil\tOH\tPaulding County\tH1\n45827\t39125\tCloverdale\tOH\tPaulding County\tH1\n45880\t39125\tPayne\tOH\tPaulding County\tH1\n45886\t39125\tScott\tOH\tPaulding County\tH1\n45851\t39125\tHaviland\tOH\tPaulding County\tH1\n45855\t39125\tLatty\tOH\tPaulding County\tH1\n43512\t39125\tDefiance\tOH\tPaulding County\tH1\n43526\t39125\tHicksville\tOH\tPaulding County\tH1\n45879\t39125\tPaulding\tOH\tPaulding County\tH1\n43556\t39125\tSherwood\tOH\tPaulding County\tH1\n43076\t39127\tThornville\tOH\tPerry County\tH1\n43777\t39127\tRoseville\tOH\tPerry County\tH1\n43148\t39127\tPleasantville\tOH\tPerry County\tH1\n43739\t39127\tGlenford\tOH\tPerry County\tH1\n43748\t39127\tJunction city\tOH\tPerry County\tH1\n43783\t39127\tSomerset\tOH\tPerry County\tH1\n43766\t39127\tNew straitsville\tOH\tPerry County\tH1\n43760\t39127\tMount perry\tOH\tPerry County\tH1\n43107\t39127\tBremen\tOH\tPerry County\tH1\n43730\t39127\tCorning\tOH\tPerry County\tH1\n43764\t39127\tNew lexington\tOH\tPerry County\tH1\n45732\t39127\tGlouster\tOH\tPerry County\tH1\n43761\t39127\tMoxahala\tOH\tPerry County\tH1\n43138\t39127\tLogan\tOH\tPerry County\tH1\n43731\t39127\tCrooksville\tOH\tPerry County\tH1\n43150\t39127\tRushville\tOH\tPerry County\tH1\n43782\t39127\tShawnee\tOH\tPerry County\tH1\n43137\t39129\tLockbourne\tOH\tPickaway County\tH1\n43126\t39129\tHarrisburg\tOH\tPickaway County\tH1\n43145\t39129\tNew holland\tOH\tPickaway County\tH1\n43115\t39129\tClarksburg\tOH\tPickaway County\tH1\n43110\t39129\tCanal winchester\tOH\tPickaway County\tH1\n43156\t39129\tTarlton\tOH\tPickaway County\tH1\n43102\t39129\tAmanda\tOH\tPickaway County\tH1\n43143\t39129\tMount sterling\tOH\tPickaway County\tH1\n43154\t39129\tStoutsville\tOH\tPickaway County\tH1\n43101\t39129\tAdelphi\tOH\tPickaway County\tH1\n43217\t39129\tColumbus\tOH\tPickaway County\tH1\n43116\t39129\tCommercial point\tOH\tPickaway County\tH1\n43117\t39129\tDerby\tOH\tPickaway County\tH1\n43103\t39129\tAshville\tOH\tPickaway County\tH1\n43113\t39129\tCircleville\tOH\tPickaway County\tH1\n43164\t39129\tWilliamsport\tOH\tPickaway County\tH1\n45644\t39129\tKingston\tOH\tPickaway County\tH1\n43135\t39129\tLaurelville\tOH\tPickaway County\tH1\n43146\t39129\tOrient\tOH\tPickaway County\tH1\n43125\t39129\tGroveport\tOH\tPickaway County\tH1\n45660\t39131\tPeebles\tOH\tPike County\tH1\n45601\t39131\tChillicothe\tOH\tPike County\tH1\n45690\t39131\tWaverly\tOH\tPike County\tH1\n45648\t39131\tLucasville\tOH\tPike County\tH1\n45642\t39131\tJasper\tOH\tPike County\tH1\n45624\t39131\tCynthiana\tOH\tPike County\tH1\n45661\t39131\tPiketon\tOH\tPike County\tH1\n45687\t39131\tWakefield\tOH\tPike County\tH1\n45133\t39131\tHillsboro\tOH\tPike County\tH1\n45671\t39131\tRarden\tOH\tPike County\tH1\n45613\t39131\tBeaver\tOH\tPike County\tH1\n45657\t39131\tOtway\tOH\tPike County\tH1\n45612\t39131\tBainbridge\tOH\tPike County\tH1\n45646\t39131\tLatham\tOH\tPike County\tH1\n44272\t39133\tRootstown\tOH\tPortage County\tH1\n44449\t39133\tNorth benton\tOH\tPortage County\tH1\n44278\t39133\tTallmadge\tOH\tPortage County\tH1\n44260\t39133\tMogadore\tOH\tPortage County\tH1\n44243\t39133\tKent\tOH\tPortage County\tH1\n44285\t39133\tWayland\tOH\tPortage County\tH1\n44242\t39133\tKent\tOH\tPortage County\tH1\n44236\t39133\tHudson\tOH\tPortage County\tH1\n44211\t39133\tBrady lake\tOH\tPortage County\tH1\n44240\t39133\tKent\tOH\tPortage County\tH1\n44241\t39133\tStreetsboro\tOH\tPortage County\tH1\n44266\t39133\tRavenna\tOH\tPortage County\t
